vi "Sync Ch Frm Id.vi"(6 "IdOrder":u16, 7 "IdPos":u16, 9 "IdCnt":u16, 10 "Channel":u8, 11 "devId":i32) -> (2 "devId out":i32, 3 "function return":i32)   [LabVIEW 2013, in "CHR34XXX.lvlib"]
doc: "DLL BOOL __stdcall CHR34XXX_Sync_Ch_LocalAddr(IN int devId,IN BYTE Channel,IN BYTE LocalAddr); DLL BOOL __stdcall CHR34XXX_Sync_Ch_SetCrc(IN int devId,IN BYTE Channel,IN BYTE CrcVal,IN BYTE CrcOrder); DLL BOOL __stdcall CHR34XXX_Sync_Ch_FrmId(IN int devId,IN BYTE Channel,IN WORD IdCnt,IN WORD IdPos,IN WORD IdOrder);"
uses:
  CHR34XXX.lvlib
  CHR34XXX.dll
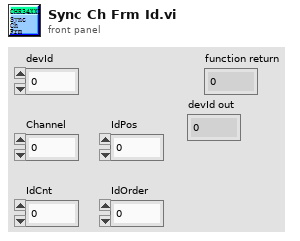
[diagram p1: front panel]
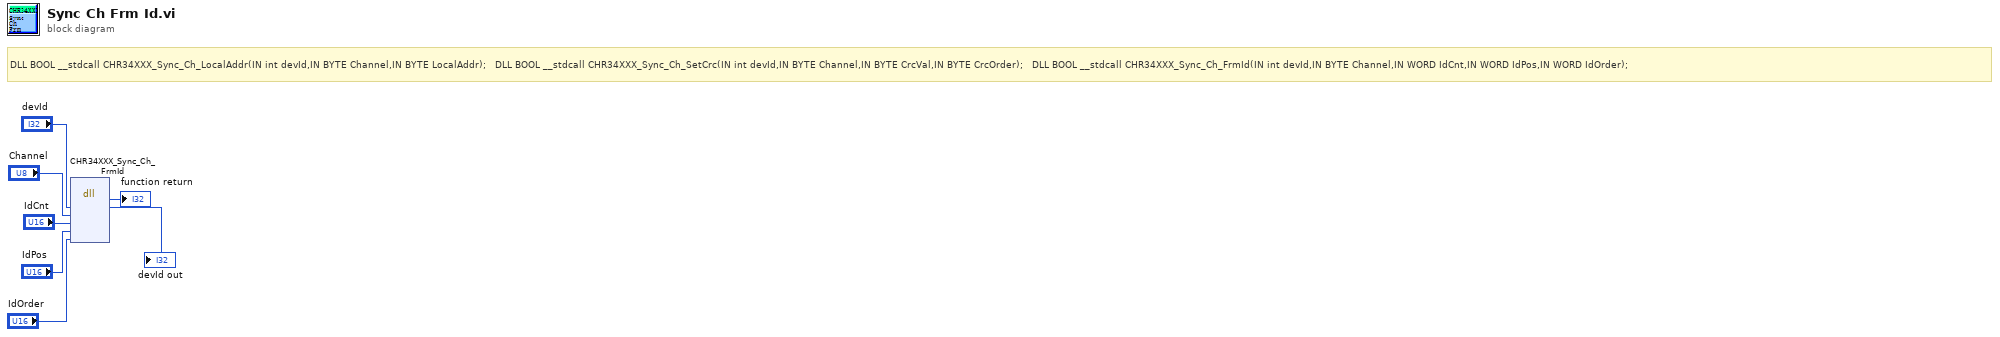
[diagram p0: block diagram]
diagram:
  # "DLL BOOL __stdcall CHR34XXX_Sync_Ch_LocalAddr(IN int devId,IN BYTE Channel,IN BYTE LocalAddr);   DLL BOOL __stdcall CHR34XXX_Sync_Ch_SetCrc(IN int devId,IN BYTE Channel,IN BYTE CrcVal,IN BYTE CrcOrder);   DLL BOOL __stdcall CHR34XXX_Sync_Ch_FrmId(IN int devId,IN BYTE Channel,IN WORD IdCnt,IN WORD IdPos,IN WORD IdOrder);"
  n1 = dll-call lib="C:/Users/Administrator/Desktop/CHR34XXX_lv/lv_lib/CHR34XXX.*" fn="CHR34XXX_Sync_Ch_FrmId"("devId"="devId", "Channel"="Channel", "IdCnt"="IdCnt", "IdPos"="IdPos", "IdOrder"="IdOrder") -> (→"function return":i32, "devId"=→"devId out":i32)  [unwired: 7 in, 2 out]
